vi "last_exp_settings_query.vi"(8 "error in (no error)":errorcluster, 11 "Small?":bool) -> (0 "error out":errorcluster, 1 "Experiment Name":string, 2 "Group Name":string, 3 "Experiment Settings":T1, 4 "Experiment ID":i64, 5 "Group ID":i64)   [LabVIEW 2013]
doc: "Displays a standard dialog box that prompts users to enter information, such as a user name and password.\n--------------------\n\nThis Express VI is configured as follows:\n\nMessage to Display to the User:Please Enter Experiment Settings Information For Database Storage.\nThe inputs are: \nNumber: Please Enter Group ID\nText Entry Box: Please Enter Tags:\nText Entry Box: Please Enter Experiment Description:"
uses:
  Public API/DisplayExperimentSetting.ctl
  <vilib>/addons/database/_DB Variant To Data/Database Variant To Data.xnode
panel:
  # "Experiment Status:"
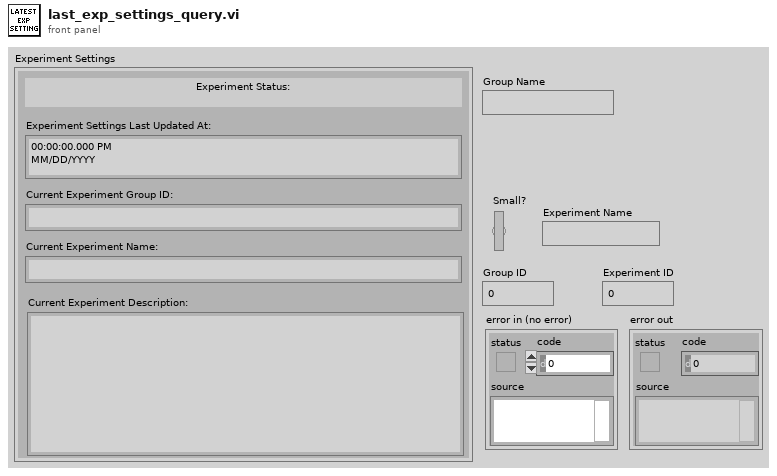
[diagram p1: front panel]
types:
  T1 = typedef "DisplayExperimentSetting.ctl" = cluster{"Current Experiment Name:":string, "Current Experiment Description:":string, "Current Experiment Group ID:":string, "Experiment Settings Last Updated At:":timestamp}
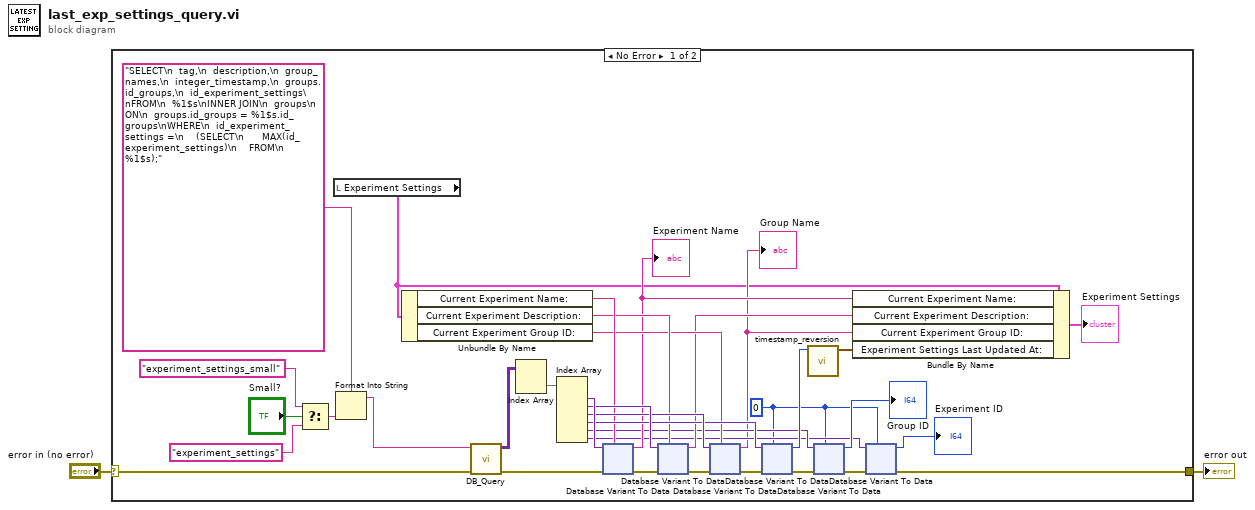
[diagram p0: block diagram]
diagram:
  n1 = case shown="No Error" "error in (no error)" {
    selector: "error in (no error)" -> [w9 w230]
    tunnel: [w6 w230] -> w1
    frame No Error {
      w14 = i64 0 ("Experiment settings ID")
      n2 = Select(t="experiment_settings_small", s="Small?", f="experiment_settings") -> (s? t:f=w12:string)
      n3 = local read "Experiment Settings"() -> (w3:T1)
      n4 = Format Into String(format string="SELECT\n  tag,\n  description,\n  group_names,\n  integer_timestamp,\n  groups.id_groups,\n  id_experiment_settings\nFROM\n  %1$s\nINNER JOIN\n  groups\n    ON\n  groups.id_groups = %1$s.id_groups\nWHERE\n  id_experiment_settings =\n    (SELECT\n      MAX(id_experiment_settings)\n    FROM\n      %1$s);" ("SQL query"), w12) -> (resulting string=w5:string)  [unwired: 2 in, 1 out]
      n5 = Unbundle By Name(w3) -> ("Current Experiment Name:"=w26:string, "Current Experiment Description:"=w24:string, "Current Experiment Group ID:"=w23:string)
      n6 = call "DB_Query.vi"("error in (no error)"=w9, "Parameterized Query"=w5) -> ("error out"=w8:errorcluster, "Results"=w7:variant[][])  [unwired: 7 in, 1 out]
      n7 = Index Array(array=w7) -> (element=w27:variant[])  [unwired: 2 in]
      n8 = Index Array(array=w27) -> (element #1=w34:variant, element #2=w33:variant, element #3=w29:variant, element #4=w28:variant, element #5=w16:variant, element #6=w15:variant)  [unwired: 6 in]
      n9 = xnode "Database Variant To Data"("database variant"=w34, "error in (no error)"=w8, "type"=w26) -> ("data"=w22:string, "error out"=w32:errorcluster)
      "Experiment Name" <- w22
      n10 = xnode "Database Variant To Data"("database variant"=w33, "error in (no error)"=w32, "type"=w24) -> ("data"=w21:string, "error out"=w31:errorcluster)
      n11 = xnode "Database Variant To Data"("database variant"=w29, "error in (no error)"=w31, "type"=w23) -> ("data"=w4:string, "error out"=w30:errorcluster)
      "Group Name" <- w4
      n12 = xnode "Database Variant To Data"("database variant"=w28, "error in (no error)"=w30, "type"=w14) -> ("data"=w25:i64, "error out"=w20:errorcluster)
      n13 = call "timestamp_reversion.vi"("Integer Timestamp"=w25) -> ("time stamp"=w37:timestamp)  [unwired: 8 in, 1 out]
      n14 = xnode "Database Variant To Data"("database variant"=w16, "error in (no error)"=w20, "type"=w14) -> ("data"=→"Group ID":i64, "error out"=w19:errorcluster)
      n15 = Bundle By Name(cluster=w3, "Current Experiment Name:"=w22, "Current Experiment Description:"=w21, "Current Experiment Group ID:"=w4, "Experiment Settings Last Updated At:"=w37) -> (→"Experiment Settings":T1)
      n16 = xnode "Database Variant To Data"("database variant"=w15, "error in (no error)"=w19, "type"=w14) -> ("data"=→"Experiment ID":i64, "error out"=w6:errorcluster)
    }
    frame Error {
    }
  }
  "error out" <- w1
